vi "SP_OEE_2_test.vi"() -> ()   [LabVIEW 2017] (continued)
                        n1462 = Transpose 2D Array(2D array=w7971) -> (transposed array=w7965:string[][])
                        n1463 = Number To Decimal String(number=w7982) -> (decimal integer string=w7977:string[])  [unwired: 1 in]
                        n1464 = Build Array(w7955) -> (w7958:string[][])
                        n1465 = Transpose 2D Array(2D array=w7958) -> (transposed array=w7964:string[][])
                      }
                      frame #7 {
                        w7985 = string[] [""]
                        n1466 = Insert Into Array(array=w7995, index (col)=1 ("disabled index (col)"), new element #1=w7985, new element #2=w7985, new element #3=w7985, new element #4=w7985, new element #5=w7985, new element #6=w7985, new element #7=w7985, new element #8=w7985, new element #9=w7986, new element #10=w7987, new element #11=w7988, new element #12=w7989) -> (w7991:string[][])  [unwired: 1 in]
                        n1467 = call "flot graph for month n year.vi"("BD Date"=w7992, "error in (no error)"=w7994, "Count total"=w7988) -> ("error out"=w7993:errorcluster, "Run-Time Status"=w7990:cluster{"Array 2":timestamp[], dbl[]})  [unwired: 7 in]
                        n1468 = local write "Run-Time Status"(w7990) -> ()
                        n1469 = local write "Table"(w7991) -> ()
                      }
                    }
                  }
                  frame "3" {
                    n1470 = flat-sequence {
                      tunnel: w8008 -> [w8122]
                      tunnel: w8007 -> [w8120]
                      tunnel: [w8106] -> w8098
                      tunnel: [w8121] -> w8097
                      tunnel: w8006 -> [_]
                      tunnel: [w8125] -> w8096
                      tunnel: [w8105] -> w8095
                      tunnel: [w8104] -> w8094
                      tunnel: [w8103] -> w8093
                      tunnel: w8005 -> [w8105]
                      tunnel: w8004 -> [w8104]
                      tunnel: ["Where BREAKDOWN_DATE between '%s'and '%s' and BREAKDOWN_STK_HOLD_ID ='%d' and  SHIFT_ID = '%d' "] -> w8092
                      tunnel: [w8103] -> w8091
                      tunnel: w8003 -> [w8099]
                      tunnel: [w8099] -> w8002
                      tunnel: w8098 -> [w8186]
                      tunnel: w8097 -> [w8188]
                      tunnel: w8096 -> [w8184]
                      tunnel: w8095 -> [w8183]
                      tunnel: w8094 -> [w8182]
                      tunnel: [w8185] -> w8090
                      tunnel: [w8187] -> w8089
                      tunnel: [w8184] -> w8088
                      tunnel: [w8174] -> w8087
                      tunnel: [w8180] -> w8086
                      tunnel: [w8183] -> w8085
                      tunnel: [w8182] -> w8084
                      tunnel: w8093 -> [w8179]
                      tunnel: [w8179] -> w8083
                      tunnel: w8092 -> [w8176]
                      tunnel: [w8176] -> w8082
                      tunnel: [w8175] -> w8081
                      tunnel: w8091 -> [w8175]
                      tunnel: w8002 -> [w8173]
                      tunnel: [w8172] -> w8001
                      tunnel: w8090 -> [w8218]
                      tunnel: w8089 -> [w8216]
                      tunnel: w8088 -> [w8221]
                      tunnel: w8087 -> [w8220]
                      tunnel: w8086 -> [w8219]
                      tunnel: w8085 -> [w8214]
                      tunnel: w8084 -> [w8213]
                      tunnel: [w8221] -> w8080
                      tunnel: [w8220] -> w8079
                      tunnel: [w8219] -> w8078
                      tunnel: [w8217] -> w8077
                      tunnel: [w8211] -> w8076
                      tunnel: [w8210] -> w8075
                      tunnel: [w8215] -> w8074
                      tunnel: [w8214] -> w8073
                      tunnel: [w8213] -> w8072
                      tunnel: w8083 -> [w8209]
                      tunnel: [w8209] -> w8071
                      tunnel: w8082 -> [w8206]
                      tunnel: [w8206] -> w8070
                      tunnel: [w8205] -> w8069
                      tunnel: w8081 -> [w8205]
                      tunnel: w8001 -> [w8204]
                      tunnel: [w8203] -> w8000
                      tunnel: w8080 -> [w8256]
                      tunnel: w8079 -> [w8255]
                      tunnel: w8078 -> [w8254]
                      tunnel: w8077 -> [w8251]
                      tunnel: w8076 -> [w8253]
                      tunnel: w8075 -> [w8252]
                      tunnel: w8074 -> [w8249]
                      tunnel: w8073 -> [w8247]
                      tunnel: w8072 -> [w8246]
                      tunnel: [w8256] -> w8068
                      tunnel: [w8255] -> w8067
                      tunnel: [w8254] -> w8066
                      tunnel: [w8253] -> w8065
                      tunnel: [w8252] -> w8064
                      tunnel: [w8250] -> w8063
                      tunnel: [w8244] -> w8062
                      tunnel: [w8243] -> w8061
                      tunnel: [w8248] -> w8060
                      tunnel: [w8247] -> w8059
                      tunnel: [w8246] -> w8058
                      tunnel: w8071 -> [w8242]
                      tunnel: [w8242] -> w8057
                      tunnel: w8070 -> [w8239]
                      tunnel: [w8239] -> w8056
                      tunnel: [w8238] -> w8055
                      tunnel: w8069 -> [w8238]
                      tunnel: w8000 -> [w8237]
                      tunnel: [w8236] -> w7999
                      tunnel: w8068 -> [w8293]
                      tunnel: w8067 -> [w8292]
                      tunnel: w8066 -> [w8291]
                      tunnel: w8065 -> [w8290]
                      tunnel: w8064 -> [w8289]
                      tunnel: w8063 -> [w8286]
                      tunnel: w8062 -> [w8288]
                      tunnel: w8061 -> [w8287]
                      tunnel: w8060 -> [w8285]
                      tunnel: w8059 -> [w8282]
                      tunnel: w8058 -> [w8281]
                      tunnel: [w8293] -> w8054
                      tunnel: [w8292] -> w8053
                      tunnel: [w8291] -> w8052
                      tunnel: [w8290] -> w8051
                      tunnel: [w8289] -> w8050
                      tunnel: [w8288] -> w8049
                      tunnel: [w8287] -> w8048
                      tunnel: [w8284] -> w8047
                      tunnel: [w8283] -> w8046
                      tunnel: [w8279] -> w8045
                      tunnel: [w8278] -> w8044
                      tunnel: [w8282] -> w8043
                      tunnel: [w8281] -> w8042
                      tunnel: w8057 -> [w8277]
                      tunnel: [w8277] -> w8041
                      tunnel: w8056 -> [w8274]
                      tunnel: [w8274] -> w8040
                      tunnel: [w8273] -> w8039
                      tunnel: w8055 -> [w8273]
                      tunnel: w7999 -> [w8272]
                      tunnel: [w8271] -> w7998
                      tunnel: w8054 -> [w8332]
                      tunnel: w8053 -> [w8331]
                      tunnel: w8052 -> [w8330]
                      tunnel: w8051 -> [w8329]
                      tunnel: w8050 -> [w8328]
                      tunnel: w8049 -> [w8327]
                      tunnel: w8048 -> [w8326]
                      tunnel: w8047 -> [w8321]
                      tunnel: w8046 -> [w8323]
                      tunnel: w8045 -> [w8325]
                      tunnel: w8044 -> [w8324]
                      tunnel: w8043 -> [w8318]
                      tunnel: w8042 -> [w8319]
                      tunnel: [w8332] -> w8038
                      tunnel: [w8331] -> w8037
                      tunnel: [w8330] -> w8036
                      tunnel: [w8329] -> w8035
                      tunnel: [w8328] -> w8034
                      tunnel: [w8327] -> w8033
                      tunnel: [w8326] -> w8032
                      tunnel: [w8325] -> w8031
                      tunnel: [w8324] -> w8030
                      tunnel: [w8322] -> w8029
                      tunnel: [w8320] -> w8028
                      tunnel: [w8316] -> w8027
                      tunnel: [w8314] -> w8026
                      tunnel: w8041 -> [w8315]
                      tunnel: w8040 -> [w8311]
                      tunnel: [w8310] -> w8025
                      tunnel: w8039 -> [w8310]
                      tunnel: w7998 -> [w8308]
                      tunnel: w8038 -> [w8359]
                      tunnel: w8037 -> [w8352]
                      tunnel: w8036 -> [w8343]
                      tunnel: w8035 -> [w8351]
                      tunnel: w8034 -> [w8341]
                      tunnel: w8033 -> [w8350]
                      tunnel: w8032 -> [w8339]
                      tunnel: w8031 -> [w8349]
                      tunnel: w8030 -> [w8337]
                      tunnel: w8029 -> [w8373]
                      tunnel: w8028 -> [w8372]
                      tunnel: w8027 -> [w8348]
                      tunnel: w8026 -> [w8335]
                      tunnel: [w8373] -> w8024
                      tunnel: [w8372] -> w8023
                      tunnel: [w8366] -> w8022
                      tunnel: [w8359] -> w8021
                      tunnel: [w8358] -> w8020
                      tunnel: [w8357] -> w8019
                      tunnel: [w8356] -> w8018
                      tunnel: [w8355] -> w8017
                      tunnel: [w8354] -> w8016
                      tunnel: [w8353] -> w8015
                      tunnel: [w8352] -> w8014
                      tunnel: [w8351] -> w8013
                      tunnel: [w8350] -> w8012
                      tunnel: [w8349] -> w8011
                      tunnel: [w8348] -> w8010
                      tunnel: [w8333] -> w8009
                      tunnel: w8025 -> [w8333]
                      tunnel: [w8386] -> _
                      tunnel: [w8382] -> _
                      tunnel: w8024 -> [w8383]
                      tunnel: w8023 -> [w8386]
                      tunnel: w8022 -> [w8377]
                      tunnel: w8021 -> [w8384]
                      tunnel: w8020 -> [_]
                      tunnel: w8019 -> [_]
                      tunnel: w8018 -> [_]
                      tunnel: w8017 -> [_]
                      tunnel: w8016 -> [w8376]
                      tunnel: w8015 -> [w8378]
                      tunnel: w8014 -> [_]
                      tunnel: w8013 -> [_]
                      tunnel: w8012 -> [_]
                      tunnel: w8011 -> [_]
                      tunnel: w8010 -> [w8375]
                      tunnel: w8009 -> [w8381]
                      frame #0 {
                        w8113 = "%Y-%m-%d" ("time format string (%c)")
                        n1471 = Decimal String To Number(string=w8099) -> (number=w8100:i32)  [unwired: 2 in, 1 out]
                        n1472 = property on="Table" class="Tbl (strict)"("Visible"=TRUE) -> ()  [unwired: 2 in, 2 out]
                        n1473 = Format Date/Time String(time format string (%c)=w8113, seconds (now)=w8105) -> (date/time string=w8114:string)  [unwired: 1 in]
                        n1474 = Format Date/Time String(time format string (%c)=w8113, seconds (now)=w8104) -> (date/time string=w8112:string)  [unwired: 1 in]
                        n1475 = Format Into String(format string="Where BREAKDOWN_DATE between '%s' and '%s' and  SHIFT_ID = '%d'  ", w8114, w8112, w8100) -> (resulting string=w8111:string)  [unwired: 2 in, 1 out]
                        n1476 = call <vilib>:"DB Tools Select Data.vi"("condition"=w8111, "error in (no error)"=w8120, "columns"=string[] ["BREAKDOWN_DATE"], "table"="STATION_1_LOG_HISTORY", "connection reference"=w8122) -> ("error out"=w8107:errorcluster, "data"=w8110:variant[][], "connection reference out"=w8121:T2)  [unwired: 1 in]
                        n1477 = property on="Table 2" class="Tbl (strict)"("Visible"=FALSE) -> ()  [unwired: 2 in, 2 out]
                        n1478 = xnode "Database Variant To Data"("database variant"=w8110, "error in (no error)"=w8107, "type"=string[][] [] ("Elements Found")) -> ("data"=w8108:string[][], "error out"=w8106:errorcluster)
                        n1479 = Index Array(array=w8108, index (col)=0 ("disabled index (col)")) -> (element=w8116:string[])  [unwired: 1 in]
                        n1480 = call "Search_1d_array_element.vi"("Count in"=string[] [] ("Elements Found"), "BD Date"=w8116, "Elements Found in"=string[] [] ("Elements Found")) -> ("Elements Found out"=w8103:string[])  [unwired: 4 in, 2 out]
                        n1481 = Build Array(w8103) -> (w8126:string[][])
                        n1482 = Transpose 2D Array(2D array=w8126) -> (transposed array=w8125:string[][])
                      }
                      frame #1 {
                        n1483 = disable-structure shown="Enabled" {
                          disable-tunnel: w8188 -> [w8199 w8201]
                          disable-tunnel: [w8198 w8201] -> w8187
                          disable-tunnel: w8186 -> [w8197 w8202]
                          disable-tunnel: [w8196 w8202] -> w8185
                          disable-tunnel: w8183 -> [w8194 _]
                          disable-tunnel: w8182 -> [w8193 _]
                          disable-tunnel: [w8192 _] -> w8181
                          disable-tunnel: [w8191 _] -> w8178
                          disable-tunnel: w8176 -> [w8190 _]
                          disable-tunnel: w8173 -> [w8189 w8200]
                          disable-tunnel: [_ w8200] -> w8172
                          frame Disabled {
                            n1484 = call "Stack_holderwise_total_bd_count_&_duration_2.vi"("Refnum in"=w8199, "BREAKDOWN_STK_HOLD_ID"=1, "condition"=w8190, "Form Date"=w8194, "To Date"=w8193, "error in (no error)"=w8197, "Shift"=w8189) -> ("Refnum out"=w8198:T2, "Count out"=w8192:string[], "appended array"=w8191:dbl[], "error out"=w8196:errorcluster)  [unwired: 5 in]
                          }
                          frame Enabled {
                          }
                        }
                        n1485 = call "NUMERIC TO STRING.vi"("appended array"=w8178) -> ("Array"=w8177:string[])  [unwired: 4 in]
                        n1486 = call "Insert_empty_element_with_zero.vi"("searched date"=w8181, "fixed date"=w8179) -> ("O/P"=w8174:string[])  [unwired: 9 in]
                        n1487 = call "Insert_empty_element_with_zero.vi"("searched date"=w8177, "fixed date"=w8179) -> ("O/P"=w8180:string[])  [unwired: 9 in]
                      }
                      frame #2 {
                        n1488 = disable-structure shown="Enabled" {
                          disable-tunnel: w8218 -> [w8232 w8234]
                          disable-tunnel: [w8231 w8234] -> w8217
                          disable-tunnel: w8216 -> [w8230 w8235]
                          disable-tunnel: [w8229 w8235] -> w8215
                          disable-tunnel: w8214 -> [w8228 _]
                          disable-tunnel: w8213 -> [w8227 _]
                          disable-tunnel: [w8226 _] -> w8212
                          disable-tunnel: [w8225 _] -> w8208
                          disable-tunnel: w8206 -> [w8224 _]
                          disable-tunnel: w8204 -> [w8222 w8233]
                          disable-tunnel: [_ w8233] -> w8203
                          frame Disabled {
                            n1489 = call "Stack_holderwise_total_bd_count_&_duration_2.vi"("Refnum in"=w8230, "BREAKDOWN_STK_HOLD_ID"=2, "condition"=w8224, "Form Date"=w8228, "To Date"=w8227, "error in (no error)"=w8232, "Shift"=w8222) -> ("Refnum out"=w8229:T2, "Count out"=w8226:string[], "appended array"=w8225:dbl[], "error out"=w8231:errorcluster)  [unwired: 5 in]
                          }
                          frame Enabled {
                          }
                        }
                        n1490 = call "Insert_empty_element_with_zero.vi"("searched date"=w8212, "fixed date"=w8209) -> ("O/P"=w8211:string[])  [unwired: 9 in]
                        n1491 = call "NUMERIC TO STRING.vi"("appended array"=w8208) -> ("Array"=w8207:string[])  [unwired: 4 in]
                        n1492 = call "Insert_empty_element_with_zero.vi"("searched date"=w8207, "fixed date"=w8209) -> ("O/P"=w8210:string[])  [unwired: 9 in]
                      }
                      frame #3 {
                        n1493 = disable-structure shown="Enabled" {
                          disable-tunnel: w8251 -> [w8267 w8269]
                          disable-tunnel: [w8266 w8269] -> w8250
                          disable-tunnel: w8249 -> [w8265 w8270]
                          disable-tunnel: [w8264 w8270] -> w8248
                          disable-tunnel: w8247 -> [w8263 _]
                          disable-tunnel: w8246 -> [w8262 _]
                          disable-tunnel: [w8261 _] -> w8245
                          disable-tunnel: [w8260 _] -> w8241
                          disable-tunnel: w8239 -> [w8259 _]
                          disable-tunnel: w8237 -> [w8257 w8268]
                          disable-tunnel: [_ w8268] -> w8236
                          frame Disabled {
                            n1494 = call "Stack_holderwise_total_bd_count_&_duration_2.vi"("Refnum in"=w8265, "BREAKDOWN_STK_HOLD_ID"=3, "condition"=w8259, "Form Date"=w8263, "To Date"=w8262, "error in (no error)"=w8267, "Shift"=w8257) -> ("Refnum out"=w8264:T2, "Count out"=w8261:string[], "appended array"=w8260:dbl[], "error out"=w8266:errorcluster)  [unwired: 5 in]
                          }
                          frame Enabled {
                          }
                        }
                        n1495 = call "Insert_empty_element_with_zero.vi"("searched date"=w8245, "fixed date"=w8242) -> ("O/P"=w8244:string[])  [unwired: 9 in]
                        n1496 = call "NUMERIC TO STRING.vi"("appended array"=w8241) -> ("Array"=w8240:string[])  [unwired: 4 in]
                        n1497 = call "Insert_empty_element_with_zero.vi"("searched date"=w8240, "fixed date"=w8242) -> ("O/P"=w8243:string[])  [unwired: 9 in]
                      }
                      frame #4 {
                        n1498 = disable-structure shown="Enabled" {
                          disable-tunnel: w8286 -> [w8304 w8307]
                          disable-tunnel: w8285 -> [w8303 w8306]
                          disable-tunnel: [w8302 w8306] -> w8284
                          disable-tunnel: [w8301 w8307] -> w8283
                          disable-tunnel: w8282 -> [w8300 _]
                          disable-tunnel: w8281 -> [w8299 _]
                          disable-tunnel: [w8298 _] -> w8280
                          disable-tunnel: [w8297 _] -> w8276
                          disable-tunnel: w8274 -> [w8296 _]
                          disable-tunnel: w8272 -> [w8294 w8305]
                          disable-tunnel: [_ w8305] -> w8271
                          frame Disabled {
                            n1499 = call "Stack_holderwise_total_bd_count_&_duration_2.vi"("Refnum in"=w8303, "BREAKDOWN_STK_HOLD_ID"=4, "condition"=w8296, "Form Date"=w8300, "To Date"=w8299, "error in (no error)"=w8304, "Shift"=w8294) -> ("Refnum out"=w8302:T2, "Count out"=w8298:string[], "appended array"=w8297:dbl[], "error out"=w8301:errorcluster)  [unwired: 5 in]
                          }
                          frame Enabled {
                          }
                        }
                        n1500 = call "Insert_empty_element_with_zero.vi"("searched date"=w8280, "fixed date"=w8277) -> ("O/P"=w8279:string[])  [unwired: 9 in]
                        n1501 = call "NUMERIC TO STRING.vi"("appended array"=w8276) -> ("Array"=w8275:string[])  [unwired: 4 in]
                        n1502 = call "Insert_empty_element_with_zero.vi"("searched date"=w8275, "fixed date"=w8277) -> ("O/P"=w8278:string[])  [unwired: 9 in]
                      }
                      frame #5 {
                        n1503 = call "Stack_holderwise_total_bd_count_&_duration_2.vi"("Refnum in"=w8321, "BREAKDOWN_STK_HOLD_ID"=5, "condition"=w8311, "Form Date"=w8318, "To Date"=w8319, "error in (no error)"=w8323, "Shift"=w8308) -> ("Refnum out"=w8320:T2, "Count out"=w8317:string[], "appended array"=w8313:dbl[], "error out"=w8322:errorcluster)  [unwired: 5 in]
                        n1504 = call "NUMERIC TO STRING.vi"("appended array"=w8313) -> ("Array"=w8312:string[])  [unwired: 4 in]
                        n1505 = call "Insert_empty_element_with_zero.vi"("searched date"=w8317, "fixed date"=w8315) -> ("O/P"=w8316:string[])  [unwired: 9 in]
                        n1506 = call "Insert_empty_element_with_zero.vi"("searched date"=w8312, "fixed date"=w8315) -> ("O/P"=w8314:string[])  [unwired: 9 in]
                      }
                      frame #6 {
                        n1507 = call "String to numeric.vi"("Array"=w8343) -> ("Array 2"=w8342:dbl[])  [unwired: 4 in]
                        n1508 = call "String to numeric.vi"("Array"=w8341) -> ("Array 2"=w8340:dbl[])  [unwired: 4 in]
                        n1509 = call "String to numeric.vi"("Array"=w8339) -> ("Array 2"=w8338:dbl[])  [unwired: 4 in]
                        n1510 = call "String to numeric.vi"("Array"=w8337) -> ("Array 2"=w8336:dbl[])  [unwired: 4 in]
                        n1511 = call "String to numeric.vi"("Array"=w8335) -> ("Array 2"=w8334:dbl[])  [unwired: 4 in]
                        n1512 = Decimal String To Number(string=w8348) -> (number=w8367:i32[])  [unwired: 2 in, 1 out]
                        n1513 = Decimal String To Number(string=w8349) -> (number=w8368:i32[])  [unwired: 2 in, 1 out]
                        n1514 = Decimal String To Number(string=w8350) -> (number=w8369:i32[])  [unwired: 2 in, 1 out]
                        n1515 = Decimal String To Number(string=w8351) -> (number=w8370:i32[])  [unwired: 2 in, 1 out]
                        n1516 = Decimal String To Number(string=w8352) -> (number=w8365:i32[])  [unwired: 2 in, 1 out]
                        n1517 = Compound Arithmetic op=ADD(w8342, w8340, w8338, w8336, w8334) -> (w8345:dbl[])
                        n1518 = Build Array(w8343) -> (w8364:string[][])
                        n1519 = Build Array(w8341) -> (w8363:string[][])
                        n1520 = Build Array(w8339) -> (w8362:string[][])
                        n1521 = Build Array(w8337) -> (w8361:string[][])
                        n1522 = Build Array(w8335) -> (w8360:string[][])
                        n1523 = Number To Fractional String(number=w8345, precision (6)=i16 2) -> (F-format string=w8344:string[])  [unwired: 2 in]
                        n1524 = Compound Arithmetic op=ADD(w8367, w8368, w8369, w8370, w8365) -> (w8371:i32[])
                        n1525 = Transpose 2D Array(2D array=w8364) -> (transposed array=w8358:string[][])
                        n1526 = Transpose 2D Array(2D array=w8363) -> (transposed array=w8357:string[][])
                        n1527 = Transpose 2D Array(2D array=w8362) -> (transposed array=w8356:string[][])
                        n1528 = Transpose 2D Array(2D array=w8361) -> (transposed array=w8355:string[][])
                        n1529 = Transpose 2D Array(2D array=w8360) -> (transposed array=w8354:string[][])
                        n1530 = Number To Decimal String(number=w8371) -> (decimal integer string=w8366:string[])  [unwired: 1 in]
                        n1531 = Build Array(w8344) -> (w8347:string[][])
                        n1532 = Transpose 2D Array(2D array=w8347) -> (transposed array=w8353:string[][])
                      }
                      frame #7 {
                        w8374 = string[] [""]
                        n1533 = Insert Into Array(array=w8384, index (col)=1 ("disabled index (col)"), new element #1=w8374, new element #2=w8374, new element #3=w8374, new element #4=w8374, new element #5=w8374, new element #6=w8374, new element #7=w8374, new element #8=w8374, new element #9=w8375, new element #10=w8376, new element #11=w8377, new element #12=w8378) -> (w8380:string[][])  [unwired: 1 in]
                        n1534 = call "flot graph for month n year.vi"("BD Date"=w8381, "error in (no error)"=w8383, "Count total"=w8377) -> ("error out"=w8382:errorcluster, "Run-Time Status"=w8379:cluster{"Array 2":timestamp[], dbl[]})  [unwired: 7 in]
                        n1535 = local write "Run-Time Status"(w8379) -> ()
                        n1536 = local write "Table"(w8380) -> ()
                      }
                    }
                  }
                  frame "1" {
                    n1537 = flat-sequence {
                      tunnel: w8397 -> [w8511]
                      tunnel: w8396 -> [w8509]
                      tunnel: [w8495] -> w8487
                      tunnel: [w8510] -> w8486
                      tunnel: w8395 -> [_]
                      tunnel: [w8514] -> w8485
                      tunnel: [w8494] -> w8484
                      tunnel: [w8493] -> w8483
                      tunnel: [w8492] -> w8482
                      tunnel: w8394 -> [w8494]
                      tunnel: w8393 -> [w8493]
                      tunnel: ["Where BREAKDOWN_DATE between '%s'and '%s' and BREAKDOWN_STK_HOLD_ID ='%d' and  SHIFT_ID = '%d' "] -> w8481
                      tunnel: [w8492] -> w8480
                      tunnel: w8392 -> [w8488]
                      tunnel: [w8488] -> w8391
                      tunnel: w8487 -> [w8575]
                      tunnel: w8486 -> [w8577]
                      tunnel: w8485 -> [w8573]
                      tunnel: w8484 -> [w8572]
                      tunnel: w8483 -> [w8571]
                      tunnel: [w8574] -> w8479
                      tunnel: [w8576] -> w8478
                      tunnel: [w8573] -> w8477
                      tunnel: [w8563] -> w8476
                      tunnel: [w8569] -> w8475
                      tunnel: [w8572] -> w8474
                      tunnel: [w8571] -> w8473
                      tunnel: w8482 -> [w8568]
                      tunnel: [w8568] -> w8472
                      tunnel: w8481 -> [w8565]
                      tunnel: [w8565] -> w8471
                      tunnel: [w8564] -> w8470
                      tunnel: w8480 -> [w8564]
                      tunnel: w8391 -> [w8562]
                      tunnel: [w8561] -> w8390
                      tunnel: w8479 -> [w8607]
                      tunnel: w8478 -> [w8605]
                      tunnel: w8477 -> [w8610]
                      tunnel: w8476 -> [w8609]
                      tunnel: w8475 -> [w8608]
                      tunnel: w8474 -> [w8603]
                      tunnel: w8473 -> [w8602]
                      tunnel: [w8610] -> w8469
                      tunnel: [w8609] -> w8468
                      tunnel: [w8608] -> w8467
                      tunnel: [w8606] -> w8466
                      tunnel: [w8600] -> w8465
                      tunnel: [w8599] -> w8464
                      tunnel: [w8604] -> w8463
                      tunnel: [w8603] -> w8462
                      tunnel: [w8602] -> w8461
                      tunnel: w8472 -> [w8598]
                      tunnel: [w8598] -> w8460
                      tunnel: w8471 -> [w8595]
                      tunnel: [w8595] -> w8459
                      tunnel: [w8594] -> w8458
                      tunnel: w8470 -> [w8594]
                      tunnel: w8390 -> [w8593]
                      tunnel: [w8592] -> w8389
                      tunnel: w8469 -> [w8645]
                      tunnel: w8468 -> [w8644]
                      tunnel: w8467 -> [w8643]
                      tunnel: w8466 -> [w8640]
                      tunnel: w8465 -> [w8642]
                      tunnel: w8464 -> [w8641]
                      tunnel: w8463 -> [w8638]
                      tunnel: w8462 -> [w8636]
                      tunnel: w8461 -> [w8635]
                      tunnel: [w8645] -> w8457
                      tunnel: [w8644] -> w8456
                      tunnel: [w8643] -> w8455
                      tunnel: [w8642] -> w8454
                      tunnel: [w8641] -> w8453
                      tunnel: [w8639] -> w8452
                      tunnel: [w8633] -> w8451
                      tunnel: [w8632] -> w8450
                      tunnel: [w8637] -> w8449
                      tunnel: [w8636] -> w8448
                      tunnel: [w8635] -> w8447
                      tunnel: w8460 -> [w8631]
                      tunnel: [w8631] -> w8446
                      tunnel: w8459 -> [w8628]
                      tunnel: [w8628] -> w8445
                      tunnel: [w8627] -> w8444
                      tunnel: w8458 -> [w8627]
                      tunnel: w8389 -> [w8626]
                      tunnel: [w8625] -> w8388
                      tunnel: w8457 -> [w8682]
                      tunnel: w8456 -> [w8681]
                      tunnel: w8455 -> [w8680]
                      tunnel: w8454 -> [w8679]
                      tunnel: w8453 -> [w8678]
                      tunnel: w8452 -> [w8675]
                      tunnel: w8451 -> [w8677]
                      tunnel: w8450 -> [w8676]
                      tunnel: w8449 -> [w8674]
                      tunnel: w8448 -> [w8671]
                      tunnel: w8447 -> [w8670]
                      tunnel: [w8682] -> w8443
                      tunnel: [w8681] -> w8442
                      tunnel: [w8680] -> w8441
                      tunnel: [w8679] -> w8440
                      tunnel: [w8678] -> w8439
                      tunnel: [w8677] -> w8438
                      tunnel: [w8676] -> w8437
                      tunnel: [w8673] -> w8436
                      tunnel: [w8672] -> w8435
                      tunnel: [w8668] -> w8434
                      tunnel: [w8667] -> w8433
                      tunnel: [w8671] -> w8432
                      tunnel: [w8670] -> w8431
                      tunnel: w8446 -> [w8666]
                      tunnel: [w8666] -> w8430
                      tunnel: w8445 -> [w8663]
                      tunnel: [w8663] -> w8429
                      tunnel: [w8662] -> w8428
                      tunnel: w8444 -> [w8662]
                      tunnel: w8388 -> [w8661]
                      tunnel: [w8660] -> w8387
                      tunnel: w8443 -> [w8721]
                      tunnel: w8442 -> [w8720]
                      tunnel: w8441 -> [w8719]
                      tunnel: w8440 -> [w8718]
                      tunnel: w8439 -> [w8717]
                      tunnel: w8438 -> [w8716]
                      tunnel: w8437 -> [w8715]
                      tunnel: w8436 -> [w8710]
                      tunnel: w8435 -> [w8712]
                      tunnel: w8434 -> [w8714]
                      tunnel: w8433 -> [w8713]
                      tunnel: w8432 -> [w8707]
                      tunnel: w8431 -> [w8708]
                      tunnel: [w8721] -> w8427
                      tunnel: [w8720] -> w8426
                      tunnel: [w8719] -> w8425
                      tunnel: [w8718] -> w8424
                      tunnel: [w8717] -> w8423
                      tunnel: [w8716] -> w8422
                      tunnel: [w8715] -> w8421
                      tunnel: [w8714] -> w8420
                      tunnel: [w8713] -> w8419
                      tunnel: [w8711] -> w8418
                      tunnel: [w8709] -> w8417
                      tunnel: [w8705] -> w8416
                      tunnel: [w8703] -> w8415
                      tunnel: w8430 -> [w8704]
                      tunnel: w8429 -> [w8700]
                      tunnel: [w8699] -> w8414
                      tunnel: w8428 -> [w8699]
                      tunnel: w8387 -> [w8697]
                      tunnel: w8427 -> [w8748]
                      tunnel: w8426 -> [w8741]
                      tunnel: w8425 -> [w8732]
                      tunnel: w8424 -> [w8740]
                      tunnel: w8423 -> [w8730]
                      tunnel: w8422 -> [w8739]
                      tunnel: w8421 -> [w8728]
                      tunnel: w8420 -> [w8738]
                      tunnel: w8419 -> [w8726]
                      tunnel: w8418 -> [w8762]
                      tunnel: w8417 -> [w8761]
                      tunnel: w8416 -> [w8737]
                      tunnel: w8415 -> [w8724]
                      tunnel: [w8762] -> w8413
                      tunnel: [w8761] -> w8412
                      tunnel: [w8755] -> w8411
                      tunnel: [w8748] -> w8410
                      tunnel: [w8747] -> w8409
                      tunnel: [w8746] -> w8408
                      tunnel: [w8745] -> w8407
                      tunnel: [w8744] -> w8406
                      tunnel: [w8743] -> w8405
                      tunnel: [w8742] -> w8404
                      tunnel: [w8741] -> w8403
                      tunnel: [w8740] -> w8402
                      tunnel: [w8739] -> w8401
                      tunnel: [w8738] -> w8400
                      tunnel: [w8737] -> w8399
                      tunnel: [w8722] -> w8398
                      tunnel: w8414 -> [w8722]
                      tunnel: [w8775] -> _
                      tunnel: [w8771] -> _
                      tunnel: w8413 -> [w8772]
                      tunnel: w8412 -> [w8775]
                      tunnel: w8411 -> [w8766]
                      tunnel: w8410 -> [w8773]
                      tunnel: w8409 -> [_]
                      tunnel: w8408 -> [_]
                      tunnel: w8407 -> [_]
                      tunnel: w8406 -> [_]
                      tunnel: w8405 -> [w8765]
                      tunnel: w8404 -> [w8767]
                      tunnel: w8403 -> [_]
                      tunnel: w8402 -> [_]
                      tunnel: w8401 -> [_]
                      tunnel: w8400 -> [_]
                      tunnel: w8399 -> [w8764]
                      tunnel: w8398 -> [w8770]
                      frame #0 {
                        w8502 = "%Y-%m-%d" ("time format string (%c)")
                        n1538 = Decimal String To Number(string=w8488) -> (number=w8489:i32)  [unwired: 2 in, 1 out]
                        n1539 = property on="Table" class="Tbl (strict)"("Visible"=TRUE) -> ()  [unwired: 2 in, 2 out]
                        n1540 = Format Date/Time String(time format string (%c)=w8502, seconds (now)=w8494) -> (date/time string=w8503:string)  [unwired: 1 in]
                        n1541 = Format Date/Time String(time format string (%c)=w8502, seconds (now)=w8493) -> (date/time string=w8501:string)  [unwired: 1 in]
                        n1542 = Format Into String(format string="Where BREAKDOWN_DATE between '%s' and '%s' and  SHIFT_ID = '%d'  ", w8503, w8501, w8489) -> (resulting string=w8500:string)  [unwired: 2 in, 1 out]
                        n1543 = call <vilib>:"DB Tools Select Data.vi"("condition"=w8500, "error in (no error)"=w8509, "columns"=string[] ["BREAKDOWN_DATE"], "table"="STATION_1_LOG_HISTORY", "connection reference"=w8511) -> ("error out"=w8496:errorcluster, "data"=w8499:variant[][], "connection reference out"=w8510:T2)  [unwired: 1 in]
                        n1544 = property on="Table 2" class="Tbl (strict)"("Visible"=FALSE) -> ()  [unwired: 2 in, 2 out]
                        n1545 = xnode "Database Variant To Data"("database variant"=w8499, "error in (no error)"=w8496, "type"=string[][] [] ("Elements Found")) -> ("data"=w8497:string[][], "error out"=w8495:errorcluster)
                        n1546 = Index Array(array=w8497, index (col)=0 ("disabled index (col)")) -> (element=w8505:string[])  [unwired: 1 in]
                        n1547 = call "Search_1d_array_element.vi"("Count in"=string[] [] ("Elements Found"), "BD Date"=w8505, "Elements Found in"=string[] [] ("Elements Found")) -> ("Elements Found out"=w8492:string[])  [unwired: 4 in, 2 out]
                        n1548 = Build Array(w8492) -> (w8515:string[][])
                        n1549 = Transpose 2D Array(2D array=w8515) -> (transposed array=w8514:string[][])
                      }
                      frame #1 {
                        n1550 = disable-structure shown="Enabled" {
                          disable-tunnel: w8577 -> [w8588 w8590]
                          disable-tunnel: [w8587 w8590] -> w8576
                          disable-tunnel: w8575 -> [w8586 w8591]
                          disable-tunnel: [w8585 w8591] -> w8574
                          disable-tunnel: w8572 -> [w8583 _]
                          disable-tunnel: w8571 -> [w8582 _]
                          disable-tunnel: [w8581 _] -> w8570
                          disable-tunnel: [w8580 _] -> w8567
                          disable-tunnel: w8565 -> [w8579 _]
                          disable-tunnel: w8562 -> [w8578 w8589]
                          disable-tunnel: [_ w8589] -> w8561
                          frame Disabled {
                            n1551 = call "Stack_holderwise_total_bd_count_&_duration_2.vi"("Refnum in"=w8588, "BREAKDOWN_STK_HOLD_ID"=1, "condition"=w8579, "Form Date"=w8583, "To Date"=w8582, "error in (no error)"=w8586, "Shift"=w8578) -> ("Refnum out"=w8587:T2, "Count out"=w8581:string[], "appended array"=w8580:dbl[], "error out"=w8585:errorcluster)  [unwired: 5 in]
                          }
                          frame Enabled {
                          }
                        }
                        n1552 = call "NUMERIC TO STRING.vi"("appended array"=w8567) -> ("Array"=w8566:string[])  [unwired: 4 in]
                        n1553 = call "Insert_empty_element_with_zero.vi"("searched date"=w8570, "fixed date"=w8568) -> ("O/P"=w8563:string[])  [unwired: 9 in]
                        n1554 = call "Insert_empty_element_with_zero.vi"("searched date"=w8566, "fixed date"=w8568) -> ("O/P"=w8569:string[])  [unwired: 9 in]
                      }
                      frame #2 {
                        n1555 = disable-structure shown="Enabled" {
                          disable-tunnel: w8607 -> [w8621 w8623]
                          disable-tunnel: [w8620 w8623] -> w8606
                          disable-tunnel: w8605 -> [w8619 w8624]
                          disable-tunnel: [w8618 w8624] -> w8604
                          disable-tunnel: w8603 -> [w8617 _]
                          disable-tunnel: w8602 -> [w8616 _]
                          disable-tunnel: [w8615 _] -> w8601
                          disable-tunnel: [w8614 _] -> w8597
                          disable-tunnel: w8595 -> [w8613 _]
                          disable-tunnel: w8593 -> [w8611 w8622]
                          disable-tunnel: [_ w8622] -> w8592
                          frame Disabled {
                            n1556 = call "Stack_holderwise_total_bd_count_&_duration_2.vi"("Refnum in"=w8619, "BREAKDOWN_STK_HOLD_ID"=2, "condition"=w8613, "Form Date"=w8617, "To Date"=w8616, "error in (no error)"=w8621, "Shift"=w8611) -> ("Refnum out"=w8618:T2, "Count out"=w8615:string[], "appended array"=w8614:dbl[], "error out"=w8620:errorcluster)  [unwired: 5 in]
                          }
                          frame Enabled {
                          }
                        }
                        n1557 = call "Insert_empty_element_with_zero.vi"("searched date"=w8601, "fixed date"=w8598) -> ("O/P"=w8600:string[])  [unwired: 9 in]
                        n1558 = call "NUMERIC TO STRING.vi"("appended array"=w8597) -> ("Array"=w8596:string[])  [unwired: 4 in]
                        n1559 = call "Insert_empty_element_with_zero.vi"("searched date"=w8596, "fixed date"=w8598) -> ("O/P"=w8599:string[])  [unwired: 9 in]
                      }
                      frame #3 {
                        n1560 = disable-structure shown="Enabled" {
                          disable-tunnel: w8640 -> [w8656 w8658]
                          disable-tunnel: [w8655 w8658] -> w8639
                          disable-tunnel: w8638 -> [w8654 w8659]
                          disable-tunnel: [w8653 w8659] -> w8637
                          disable-tunnel: w8636 -> [w8652 _]
                          disable-tunnel: w8635 -> [w8651 _]
                          disable-tunnel: [w8650 _] -> w8634
                          disable-tunnel: [w8649 _] -> w8630
                          disable-tunnel: w8628 -> [w8648 _]
                          disable-tunnel: w8626 -> [w8646 w8657]
                          disable-tunnel: [_ w8657] -> w8625
                          frame Disabled {
                            n1561 = call "Stack_holderwise_total_bd_count_&_duration_2.vi"("Refnum in"=w8654, "BREAKDOWN_STK_HOLD_ID"=3, "condition"=w8648, "Form Date"=w8652, "To Date"=w8651, "error in (no error)"=w8656, "Shift"=w8646) -> ("Refnum out"=w8653:T2, "Count out"=w8650:string[], "appended array"=w8649:dbl[], "error out"=w8655:errorcluster)  [unwired: 5 in]
                          }
                          frame Enabled {
                          }
                        }
                        n1562 = call "Insert_empty_element_with_zero.vi"("searched date"=w8634, "fixed date"=w8631) -> ("O/P"=w8633:string[])  [unwired: 9 in]
                        n1563 = call "NUMERIC TO STRING.vi"("appended array"=w8630) -> ("Array"=w8629:string[])  [unwired: 4 in]
                        n1564 = call "Insert_empty_element_with_zero.vi"("searched date"=w8629, "fixed date"=w8631) -> ("O/P"=w8632:string[])  [unwired: 9 in]
                      }
                      frame #4 {
                        n1565 = disable-structure shown="Enabled" {
                          disable-tunnel: w8675 -> [w8693 w8696]
                          disable-tunnel: w8674 -> [w8692 w8695]
                          disable-tunnel: [w8691 w8695] -> w8673
                          disable-tunnel: [w8690 w8696] -> w8672
                          disable-tunnel: w8671 -> [w8689 _]
                          disable-tunnel: w8670 -> [w8688 _]
                          disable-tunnel: [w8687 _] -> w8669
                          disable-tunnel: [w8686 _] -> w8665
                          disable-tunnel: w8663 -> [w8685 _]
                          disable-tunnel: w8661 -> [w8683 w8694]
                          disable-tunnel: [_ w8694] -> w8660
                          frame Disabled {
                            n1566 = call "Stack_holderwise_total_bd_count_&_duration_2.vi"("Refnum in"=w8692, "BREAKDOWN_STK_HOLD_ID"=4, "condition"=w8685, "Form Date"=w8689, "To Date"=w8688, "error in (no error)"=w8693, "Shift"=w8683) -> ("Refnum out"=w8691:T2, "Count out"=w8687:string[], "appended array"=w8686:dbl[], "error out"=w8690:errorcluster)  [unwired: 5 in]
                          }
                          frame Enabled {
                          }
                        }
                        n1567 = call "Insert_empty_element_with_zero.vi"("searched date"=w8669, "fixed date"=w8666) -> ("O/P"=w8668:string[])  [unwired: 9 in]
                        n1568 = call "NUMERIC TO STRING.vi"("appended array"=w8665) -> ("Array"=w8664:string[])  [unwired: 4 in]
                        n1569 = call "Insert_empty_element_with_zero.vi"("searched date"=w8664, "fixed date"=w8666) -> ("O/P"=w8667:string[])  [unwired: 9 in]
                      }
                      frame #5 {
                        n1570 = call "Stack_holderwise_total_bd_count_&_duration_2.vi"("Refnum in"=w8710, "BREAKDOWN_STK_HOLD_ID"=5, "condition"=w8700, "Form Date"=w8707, "To Date"=w8708, "error in (no error)"=w8712, "Shift"=w8697) -> ("Refnum out"=w8709:T2, "Count out"=w8706:string[], "appended array"=w8702:dbl[], "error out"=w8711:errorcluster)  [unwired: 5 in]
                        n1571 = call "NUMERIC TO STRING.vi"("appended array"=w8702) -> ("Array"=w8701:string[])  [unwired: 4 in]
                        n1572 = call "Insert_empty_element_with_zero.vi"("searched date"=w8706, "fixed date"=w8704) -> ("O/P"=w8705:string[])  [unwired: 9 in]
                        n1573 = call "Insert_empty_element_with_zero.vi"("searched date"=w8701, "fixed date"=w8704) -> ("O/P"=w8703:string[])  [unwired: 9 in]
                      }
                      frame #6 {
                        n1574 = call "String to numeric.vi"("Array"=w8732) -> ("Array 2"=w8731:dbl[])  [unwired: 4 in]
                        n1575 = call "String to numeric.vi"("Array"=w8730) -> ("Array 2"=w8729:dbl[])  [unwired: 4 in]
                        n1576 = call "String to numeric.vi"("Array"=w8728) -> ("Array 2"=w8727:dbl[])  [unwired: 4 in]
                        n1577 = call "String to numeric.vi"("Array"=w8726) -> ("Array 2"=w8725:dbl[])  [unwired: 4 in]
                        n1578 = call "String to numeric.vi"("Array"=w8724) -> ("Array 2"=w8723:dbl[])  [unwired: 4 in]
                        n1579 = Decimal String To Number(string=w8737) -> (number=w8756:i32[])  [unwired: 2 in, 1 out]
                        n1580 = Decimal String To Number(string=w8738) -> (number=w8757:i32[])  [unwired: 2 in, 1 out]
                        n1581 = Decimal String To Number(string=w8739) -> (number=w8758:i32[])  [unwired: 2 in, 1 out]
                        n1582 = Decimal String To Number(string=w8740) -> (number=w8759:i32[])  [unwired: 2 in, 1 out]
                        n1583 = Decimal String To Number(string=w8741) -> (number=w8754:i32[])  [unwired: 2 in, 1 out]
                        n1584 = Compound Arithmetic op=ADD(w8731, w8729, w8727, w8725, w8723) -> (w8734:dbl[])
                        n1585 = Build Array(w8732) -> (w8753:string[][])
                        n1586 = Build Array(w8730) -> (w8752:string[][])
                        n1587 = Build Array(w8728) -> (w8751:string[][])
                        n1588 = Build Array(w8726) -> (w8750:string[][])
                        n1589 = Build Array(w8724) -> (w8749:string[][])
                        n1590 = Number To Fractional String(number=w8734, precision (6)=i16 2) -> (F-format string=w8733:string[])  [unwired: 2 in]
                        n1591 = Compound Arithmetic op=ADD(w8756, w8757, w8758, w8759, w8754) -> (w8760:i32[])
                        n1592 = Transpose 2D Array(2D array=w8753) -> (transposed array=w8747:string[][])
                        n1593 = Transpose 2D Array(2D array=w8752) -> (transposed array=w8746:string[][])
                        n1594 = Transpose 2D Array(2D array=w8751) -> (transposed array=w8745:string[][])
                        n1595 = Transpose 2D Array(2D array=w8750) -> (transposed array=w8744:string[][])
                        n1596 = Transpose 2D Array(2D array=w8749) -> (transposed array=w8743:string[][])
                        n1597 = Number To Decimal String(number=w8760) -> (decimal integer string=w8755:string[])  [unwired: 1 in]
                        n1598 = Build Array(w8733) -> (w8736:string[][])
                        n1599 = Transpose 2D Array(2D array=w8736) -> (transposed array=w8742:string[][])
                      }
                      frame #7 {
                        w8763 = string[] [""]
                        n1600 = Insert Into Array(array=w8773, index (col)=1 ("disabled index (col)"), new element #1=w8763, new element #2=w8763, new element #3=w8763, new element #4=w8763, new element #5=w8763, new element #6=w8763, new element #7=w8763, new element #8=w8763, new element #9=w8764, new element #10=w8765, new element #11=w8766, new element #12=w8767) -> (w8769:string[][])  [unwired: 1 in]
                        n1601 = call "flot graph for month n year.vi"("BD Date"=w8770, "error in (no error)"=w8772, "Count total"=w8766) -> ("error out"=w8771:errorcluster, "Run-Time Status"=w8768:cluster{"Array 2":timestamp[], dbl[]})  [unwired: 7 in]
                        n1602 = local write "Run-Time Status"(w8768) -> ()
                        n1603 = local write "Table"(w8769) -> ()
                      }
                    }
                  }
                  frame "2" {
                    n1604 = flat-sequence {
                      tunnel: w8786 -> [w8900]
                      tunnel: w8785 -> [w8898]
                      tunnel: [w8884] -> w8876
                      tunnel: [w8899] -> w8875
                      tunnel: w8784 -> [_]
                      tunnel: [w8903] -> w8874
                      tunnel: [w8883] -> w8873
                      tunnel: [w8882] -> w8872
                      tunnel: [w8881] -> w8871
                      tunnel: w8783 -> [w8883]
                      tunnel: w8782 -> [w8882]
                      tunnel: ["Where BREAKDOWN_DATE between '%s'and '%s' and BREAKDOWN_STK_HOLD_ID ='%d' and  SHIFT_ID = '%d' "] -> w8870
                      tunnel: [w8881] -> w8869
                      tunnel: w8781 -> [w8877]
                      tunnel: [w8877] -> w8780
                      tunnel: w8876 -> [w8964]
                      tunnel: w8875 -> [w8966]
                      tunnel: w8874 -> [w8962]
                      tunnel: w8873 -> [w8961]
                      tunnel: w8872 -> [w8960]
                      tunnel: [w8963] -> w8868
                      tunnel: [w8965] -> w8867
                      tunnel: [w8962] -> w8866
                      tunnel: [w8952] -> w8865
                      tunnel: [w8958] -> w8864
                      tunnel: [w8961] -> w8863
                      tunnel: [w8960] -> w8862
                      tunnel: w8871 -> [w8957]
                      tunnel: [w8957] -> w8861
                      tunnel: w8870 -> [w8954]
                      tunnel: [w8954] -> w8860
                      tunnel: [w8953] -> w8859
                      tunnel: w8869 -> [w8953]
                      tunnel: w8780 -> [w8951]
                      tunnel: [w8950] -> w8779
                      tunnel: w8868 -> [w8996]
                      tunnel: w8867 -> [w8994]
                      tunnel: w8866 -> [w8999]
                      tunnel: w8865 -> [w8998]
                      tunnel: w8864 -> [w8997]
                      tunnel: w8863 -> [w8992]
                      tunnel: w8862 -> [w8991]
                      tunnel: [w8999] -> w8858
                      tunnel: [w8998] -> w8857
                      tunnel: [w8997] -> w8856
                      tunnel: [w8995] -> w8855
                      tunnel: [w8989] -> w8854
                      tunnel: [w8988] -> w8853
                      tunnel: [w8993] -> w8852
                      tunnel: [w8992] -> w8851
                      tunnel: [w8991] -> w8850
                      tunnel: w8861 -> [w8987]
                      tunnel: [w8987] -> w8849
                      tunnel: w8860 -> [w8984]
                      tunnel: [w8984] -> w8848
                      tunnel: [w8983] -> w8847
                      tunnel: w8859 -> [w8983]
                      tunnel: w8779 -> [w8982]
                      tunnel: [w8981] -> w8778
                      tunnel: w8858 -> [w9034]
                      tunnel: w8857 -> [w9033]
                      tunnel: w8856 -> [w9032]
                      tunnel: w8855 -> [w9029]
                      tunnel: w8854 -> [w9031]
                      tunnel: w8853 -> [w9030]
                      tunnel: w8852 -> [w9027]
                      tunnel: w8851 -> [w9025]
                      tunnel: w8850 -> [w9024]
                      tunnel: [w9034] -> w8846
                      tunnel: [w9033] -> w8845
                      tunnel: [w9032] -> w8844
                      tunnel: [w9031] -> w8843
                      tunnel: [w9030] -> w8842
                      tunnel: [w9028] -> w8841
                      tunnel: [w9022] -> w8840
                      tunnel: [w9021] -> w8839
                      tunnel: [w9026] -> w8838
                      tunnel: [w9025] -> w8837
                      tunnel: [w9024] -> w8836
                      tunnel: w8849 -> [w9020]
                      tunnel: [w9020] -> w8835
                      tunnel: w8848 -> [w9017]
                      tunnel: [w9017] -> w8834
                      tunnel: [w9016] -> w8833
                      tunnel: w8847 -> [w9016]
                      tunnel: w8778 -> [w9015]
                      tunnel: [w9014] -> w8777
                      tunnel: w8846 -> [w9071]
                      tunnel: w8845 -> [w9070]
                      tunnel: w8844 -> [w9069]
                      tunnel: w8843 -> [w9068]
                      tunnel: w8842 -> [w9067]
                      tunnel: w8841 -> [w9064]
                      tunnel: w8840 -> [w9066]
                      tunnel: w8839 -> [w9065]
                      tunnel: w8838 -> [w9063]
                      tunnel: w8837 -> [w9060]
                      tunnel: w8836 -> [w9059]
                      tunnel: [w9071] -> w8832
                      tunnel: [w9070] -> w8831
                      tunnel: [w9069] -> w8830
                      tunnel: [w9068] -> w8829
                      tunnel: [w9067] -> w8828
                      tunnel: [w9066] -> w8827
                      tunnel: [w9065] -> w8826
                      tunnel: [w9062] -> w8825
                      tunnel: [w9061] -> w8824
                      tunnel: [w9057] -> w8823
                      tunnel: [w9056] -> w8822
                      tunnel: [w9060] -> w8821
                      tunnel: [w9059] -> w8820
                      tunnel: w8835 -> [w9055]
                      tunnel: [w9055] -> w8819
                      tunnel: w8834 -> [w9052]
                      tunnel: [w9052] -> w8818
                      tunnel: [w9051] -> w8817
                      tunnel: w8833 -> [w9051]
                      tunnel: w8777 -> [w9050]
                      tunnel: [w9049] -> w8776
                      tunnel: w8832 -> [w9110]
                      tunnel: w8831 -> [w9109]
                      tunnel: w8830 -> [w9108]
                      tunnel: w8829 -> [w9107]
                      tunnel: w8828 -> [w9106]
                      tunnel: w8827 -> [w9105]
                      tunnel: w8826 -> [w9104]
                      tunnel: w8825 -> [w9099]
                      tunnel: w8824 -> [w9101]
                      tunnel: w8823 -> [w9103]
                      tunnel: w8822 -> [w9102]
                      tunnel: w8821 -> [w9096]
                      tunnel: w8820 -> [w9097]
                      tunnel: [w9110] -> w8816
                      tunnel: [w9109] -> w8815
                      tunnel: [w9108] -> w8814
                      tunnel: [w9107] -> w8813
                      tunnel: [w9106] -> w8812
                      tunnel: [w9105] -> w8811
                      tunnel: [w9104] -> w8810
                      tunnel: [w9103] -> w8809
                      tunnel: [w9102] -> w8808
                      tunnel: [w9100] -> w8807
                      tunnel: [w9098] -> w8806
                      tunnel: [w9094] -> w8805
                      tunnel: [w9092] -> w8804
                      tunnel: w8819 -> [w9093]
                      tunnel: w8818 -> [w9089]
                      tunnel: [w9088] -> w8803
                      tunnel: w8817 -> [w9088]
                      tunnel: w8776 -> [w9086]
                      tunnel: w8816 -> [w9137]
                      tunnel: w8815 -> [w9130]
                      tunnel: w8814 -> [w9121]
                      tunnel: w8813 -> [w9129]
                      tunnel: w8812 -> [w9119]
                      tunnel: w8811 -> [w9128]
                      tunnel: w8810 -> [w9117]
                      tunnel: w8809 -> [w9127]
                      tunnel: w8808 -> [w9115]
                      tunnel: w8807 -> [w9151]
                      tunnel: w8806 -> [w9150]
                      tunnel: w8805 -> [w9126]
                      tunnel: w8804 -> [w9113]
                      tunnel: [w9151] -> w8802
                      tunnel: [w9150] -> w8801
                      tunnel: [w9144] -> w8800
                      tunnel: [w9137] -> w8799
                      tunnel: [w9136] -> w8798
                      tunnel: [w9135] -> w8797
                      tunnel: [w9134] -> w8796
                      tunnel: [w9133] -> w8795
                      tunnel: [w9132] -> w8794
                      tunnel: [w9131] -> w8793
                      tunnel: [w9130] -> w8792
                      tunnel: [w9129] -> w8791
                      tunnel: [w9128] -> w8790
                      tunnel: [w9127] -> w8789
                      tunnel: [w9126] -> w8788
                      tunnel: [w9111] -> w8787
                      tunnel: w8803 -> [w9111]
                      tunnel: [w9164] -> _
                      tunnel: [w9160] -> _
                      tunnel: w8802 -> [w9161]
                      tunnel: w8801 -> [w9164]
                      tunnel: w8800 -> [w9155]
                      tunnel: w8799 -> [w9162]
                      tunnel: w8798 -> [_]
                      tunnel: w8797 -> [_]
                      tunnel: w8796 -> [_]
                      tunnel: w8795 -> [_]
                      tunnel: w8794 -> [w9154]
                      tunnel: w8793 -> [w9156]
                      tunnel: w8792 -> [_]
                      tunnel: w8791 -> [_]
                      tunnel: w8790 -> [_]
                      tunnel: w8789 -> [_]
                      tunnel: w8788 -> [w9153]
                      tunnel: w8787 -> [w9159]
                      frame #0 {
                        w8891 = "%Y-%m-%d" ("time format string (%c)")
                        n1605 = Decimal String To Number(string=w8877) -> (number=w8878:i32)  [unwired: 2 in, 1 out]
                        n1606 = property on="Table" class="Tbl (strict)"("Visible"=TRUE) -> ()  [unwired: 2 in, 2 out]
                        n1607 = Format Date/Time String(time format string (%c)=w8891, seconds (now)=w8883) -> (date/time string=w8892:string)  [unwired: 1 in]
                        n1608 = Format Date/Time String(time format string (%c)=w8891, seconds (now)=w8882) -> (date/time string=w8890:string)  [unwired: 1 in]
                        n1609 = Format Into String(format string="Where BREAKDOWN_DATE between '%s' and '%s' and  SHIFT_ID = '%d'  ", w8892, w8890, w8878) -> (resulting string=w8889:string)  [unwired: 2 in, 1 out]
                        n1610 = call <vilib>:"DB Tools Select Data.vi"("condition"=w8889, "error in (no error)"=w8898, "columns"=string[] ["BREAKDOWN_DATE"], "table"="STATION_1_LOG_HISTORY", "connection reference"=w8900) -> ("error out"=w8885:errorcluster, "data"=w8888:variant[][], "connection reference out"=w8899:T2)  [unwired: 1 in]
                        n1611 = property on="Table 2" class="Tbl (strict)"("Visible"=FALSE) -> ()  [unwired: 2 in, 2 out]
                        n1612 = xnode "Database Variant To Data"("database variant"=w8888, "error in (no error)"=w8885, "type"=string[][] [] ("Elements Found")) -> ("data"=w8886:string[][], "error out"=w8884:errorcluster)
                        n1613 = Index Array(array=w8886, index (col)=0 ("disabled index (col)")) -> (element=w8894:string[])  [unwired: 1 in]
                        n1614 = call "Search_1d_array_element.vi"("Count in"=string[] [] ("Elements Found"), "BD Date"=w8894, "Elements Found in"=string[] [] ("Elements Found")) -> ("Elements Found out"=w8881:string[])  [unwired: 4 in, 2 out]
                        n1615 = Build Array(w8881) -> (w8904:string[][])
                        n1616 = Transpose 2D Array(2D array=w8904) -> (transposed array=w8903:string[][])
                      }
                      frame #1 {
                        n1617 = disable-structure shown="Enabled" {
                          disable-tunnel: w8966 -> [w8977 w8979]
                          disable-tunnel: [w8976 w8979] -> w8965
                          disable-tunnel: w8964 -> [w8975 w8980]
                          disable-tunnel: [w8974 w8980] -> w8963
                          disable-tunnel: w8961 -> [w8972 _]
                          disable-tunnel: w8960 -> [w8971 _]
                          disable-tunnel: [w8970 _] -> w8959
                          disable-tunnel: [w8969 _] -> w8956
                          disable-tunnel: w8954 -> [w8968 _]
                          disable-tunnel: w8951 -> [w8967 w8978]
                          disable-tunnel: [_ w8978] -> w8950
                          frame Disabled {
                            n1618 = call "Stack_holderwise_total_bd_count_&_duration_2.vi"("Refnum in"=w8977, "BREAKDOWN_STK_HOLD_ID"=1, "condition"=w8968, "Form Date"=w8972, "To Date"=w8971, "error in (no error)"=w8975, "Shift"=w8967) -> ("Refnum out"=w8976:T2, "Count out"=w8970:string[], "appended array"=w8969:dbl[], "error out"=w8974:errorcluster)  [unwired: 5 in]
                          }
                          frame Enabled {
                          }
                        }
                        n1619 = call "NUMERIC TO STRING.vi"("appended array"=w8956) -> ("Array"=w8955:string[])  [unwired: 4 in]
                        n1620 = call "Insert_empty_element_with_zero.vi"("searched date"=w8959, "fixed date"=w8957) -> ("O/P"=w8952:string[])  [unwired: 9 in]
                        n1621 = call "Insert_empty_element_with_zero.vi"("searched date"=w8955, "fixed date"=w8957) -> ("O/P"=w8958:string[])  [unwired: 9 in]
                      }
                      frame #2 {
                        n1622 = disable-structure shown="Enabled" {
                          disable-tunnel: w8996 -> [w9010 w9012]
                          disable-tunnel: [w9009 w9012] -> w8995
                          disable-tunnel: w8994 -> [w9008 w9013]
                          disable-tunnel: [w9007 w9013] -> w8993
                          disable-tunnel: w8992 -> [w9006 _]
                          disable-tunnel: w8991 -> [w9005 _]
                          disable-tunnel: [w9004 _] -> w8990
                          disable-tunnel: [w9003 _] -> w8986
                          disable-tunnel: w8984 -> [w9002 _]
                          disable-tunnel: w8982 -> [w9000 w9011]
                          disable-tunnel: [_ w9011] -> w8981
                          frame Disabled {
                            n1623 = call "Stack_holderwise_total_bd_count_&_duration_2.vi"("Refnum in"=w9008, "BREAKDOWN_STK_HOLD_ID"=2, "condition"=w9002, "Form Date"=w9006, "To Date"=w9005, "error in (no error)"=w9010, "Shift"=w9000) -> ("Refnum out"=w9007:T2, "Count out"=w9004:string[], "appended array"=w9003:dbl[], "error out"=w9009:errorcluster)  [unwired: 5 in]
                          }
                          frame Enabled {
                          }
                        }
                        n1624 = call "Insert_empty_element_with_zero.vi"("searched date"=w8990, "fixed date"=w8987) -> ("O/P"=w8989:string[])  [unwired: 9 in]
                        n1625 = call "NUMERIC TO STRING.vi"("appended array"=w8986) -> ("Array"=w8985:string[])  [unwired: 4 in]
                        n1626 = call "Insert_empty_element_with_zero.vi"("searched date"=w8985, "fixed date"=w8987) -> ("O/P"=w8988:string[])  [unwired: 9 in]
                      }
                      frame #3 {
                        n1627 = disable-structure shown="Enabled" {
                          disable-tunnel: w9029 -> [w9045 w9047]
                          disable-tunnel: [w9044 w9047] -> w9028
                          disable-tunnel: w9027 -> [w9043 w9048]
                          disable-tunnel: [w9042 w9048] -> w9026
                          disable-tunnel: w9025 -> [w9041 _]
                          disable-tunnel: w9024 -> [w9040 _]
                          disable-tunnel: [w9039 _] -> w9023
                          disable-tunnel: [w9038 _] -> w9019
                          disable-tunnel: w9017 -> [w9037 _]
                          disable-tunnel: w9015 -> [w9035 w9046]
                          disable-tunnel: [_ w9046] -> w9014
                          frame Disabled {
                            n1628 = call "Stack_holderwise_total_bd_count_&_duration_2.vi"("Refnum in"=w9043, "BREAKDOWN_STK_HOLD_ID"=3, "condition"=w9037, "Form Date"=w9041, "To Date"=w9040, "error in (no error)"=w9045, "Shift"=w9035) -> ("Refnum out"=w9042:T2, "Count out"=w9039:string[], "appended array"=w9038:dbl[], "error out"=w9044:errorcluster)  [unwired: 5 in]
                          }
                          frame Enabled {
                          }
                        }
                        n1629 = call "Insert_empty_element_with_zero.vi"("searched date"=w9023, "fixed date"=w9020) -> ("O/P"=w9022:string[])  [unwired: 9 in]
                        n1630 = call "NUMERIC TO STRING.vi"("appended array"=w9019) -> ("Array"=w9018:string[])  [unwired: 4 in]
                        n1631 = call "Insert_empty_element_with_zero.vi"("searched date"=w9018, "fixed date"=w9020) -> ("O/P"=w9021:string[])  [unwired: 9 in]
                      }
                      frame #4 {
                        n1632 = disable-structure shown="Enabled" {
                          disable-tunnel: w9064 -> [w9082 w9085]
                          disable-tunnel: w9063 -> [w9081 w9084]
                          disable-tunnel: [w9080 w9084] -> w9062
                          disable-tunnel: [w9079 w9085] -> w9061
                          disable-tunnel: w9060 -> [w9078 _]
                          disable-tunnel: w9059 -> [w9077 _]
                          disable-tunnel: [w9076 _] -> w9058
                          disable-tunnel: [w9075 _] -> w9054
                          disable-tunnel: w9052 -> [w9074 _]
                          disable-tunnel: w9050 -> [w9072 w9083]
                          disable-tunnel: [_ w9083] -> w9049
                          frame Disabled {
                            n1633 = call "Stack_holderwise_total_bd_count_&_duration_2.vi"("Refnum in"=w9081, "BREAKDOWN_STK_HOLD_ID"=4, "condition"=w9074, "Form Date"=w9078, "To Date"=w9077, "error in (no error)"=w9082, "Shift"=w9072) -> ("Refnum out"=w9080:T2, "Count out"=w9076:string[], "appended array"=w9075:dbl[], "error out"=w9079:errorcluster)  [unwired: 5 in]
                          }
                          frame Enabled {
                          }
                        }
                        n1634 = call "Insert_empty_element_with_zero.vi"("searched date"=w9058, "fixed date"=w9055) -> ("O/P"=w9057:string[])  [unwired: 9 in]
                        n1635 = call "NUMERIC TO STRING.vi"("appended array"=w9054) -> ("Array"=w9053:string[])  [unwired: 4 in]
                        n1636 = call "Insert_empty_element_with_zero.vi"("searched date"=w9053, "fixed date"=w9055) -> ("O/P"=w9056:string[])  [unwired: 9 in]
                      }
                      frame #5 {
                        n1637 = call "Stack_holderwise_total_bd_count_&_duration_2.vi"("Refnum in"=w9099, "BREAKDOWN_STK_HOLD_ID"=5, "condition"=w9089, "Form Date"=w9096, "To Date"=w9097, "error in (no error)"=w9101, "Shift"=w9086) -> ("Refnum out"=w9098:T2, "Count out"=w9095:string[], "appended array"=w9091:dbl[], "error out"=w9100:errorcluster)  [unwired: 5 in]
                        n1638 = call "NUMERIC TO STRING.vi"("appended array"=w9091) -> ("Array"=w9090:string[])  [unwired: 4 in]
                        n1639 = call "Insert_empty_element_with_zero.vi"("searched date"=w9095, "fixed date"=w9093) -> ("O/P"=w9094:string[])  [unwired: 9 in]
                        n1640 = call "Insert_empty_element_with_zero.vi"("searched date"=w9090, "fixed date"=w9093) -> ("O/P"=w9092:string[])  [unwired: 9 in]
                      }
                      frame #6 {
                        n1641 = call "String to numeric.vi"("Array"=w9121) -> ("Array 2"=w9120:dbl[])  [unwired: 4 in]
                        n1642 = call "String to numeric.vi"("Array"=w9119) -> ("Array 2"=w9118:dbl[])  [unwired: 4 in]
                        n1643 = call "String to numeric.vi"("Array"=w9117) -> ("Array 2"=w9116:dbl[])  [unwired: 4 in]
                        n1644 = call "String to numeric.vi"("Array"=w9115) -> ("Array 2"=w9114:dbl[])  [unwired: 4 in]
                        n1645 = call "String to numeric.vi"("Array"=w9113) -> ("Array 2"=w9112:dbl[])  [unwired: 4 in]
                        n1646 = Decimal String To Number(string=w9126) -> (number=w9145:i32[])  [unwired: 2 in, 1 out]
                        n1647 = Decimal String To Number(string=w9127) -> (number=w9146:i32[])  [unwired: 2 in, 1 out]
                        n1648 = Decimal String To Number(string=w9128) -> (number=w9147:i32[])  [unwired: 2 in, 1 out]
                        n1649 = Decimal String To Number(string=w9129) -> (number=w9148:i32[])  [unwired: 2 in, 1 out]
                        n1650 = Decimal String To Number(string=w9130) -> (number=w9143:i32[])  [unwired: 2 in, 1 out]
                        n1651 = Compound Arithmetic op=ADD(w9120, w9118, w9116, w9114, w9112) -> (w9123:dbl[])
                        n1652 = Build Array(w9121) -> (w9142:string[][])
                        n1653 = Build Array(w9119) -> (w9141:string[][])
                        n1654 = Build Array(w9117) -> (w9140:string[][])
                        n1655 = Build Array(w9115) -> (w9139:string[][])
                        n1656 = Build Array(w9113) -> (w9138:string[][])
                        n1657 = Number To Fractional String(number=w9123, precision (6)=i16 2) -> (F-format string=w9122:string[])  [unwired: 2 in]
                        n1658 = Compound Arithmetic op=ADD(w9145, w9146, w9147, w9148, w9143) -> (w9149:i32[])
                        n1659 = Transpose 2D Array(2D array=w9142) -> (transposed array=w9136:string[][])
                        n1660 = Transpose 2D Array(2D array=w9141) -> (transposed array=w9135:string[][])
                        n1661 = Transpose 2D Array(2D array=w9140) -> (transposed array=w9134:string[][])
                        n1662 = Transpose 2D Array(2D array=w9139) -> (transposed array=w9133:string[][])
                        n1663 = Transpose 2D Array(2D array=w9138) -> (transposed array=w9132:string[][])
                        n1664 = Number To Decimal String(number=w9149) -> (decimal integer string=w9144:string[])  [unwired: 1 in]
                        n1665 = Build Array(w9122) -> (w9125:string[][])
                        n1666 = Transpose 2D Array(2D array=w9125) -> (transposed array=w9131:string[][])
                      }
                      frame #7 {
